vi "Display Right Click Menu.vi"(5 "Coords":T1, 7 "Tbl Refnum":refnum<vi>, 8 "error in (no error)":errorcluster, 9 "Menu Reference":refnum<k9>, 10 "Sync Notifier":refnum<notifier>, 11 "UserInterface in":refnum<class "UserInterface.lvclass">) -> (0 "error out":errorcluster)   [LabVIEW 2016, in "UserInterface.lvlib" / "UserInterface.lvclass"]
uses:
  UserInterface.lvclass
  <vilib>/Utility/miscctls.llb/LVPoint32TypeDef.ctl
  UserInterface.lvclass/UserInterface.ctl
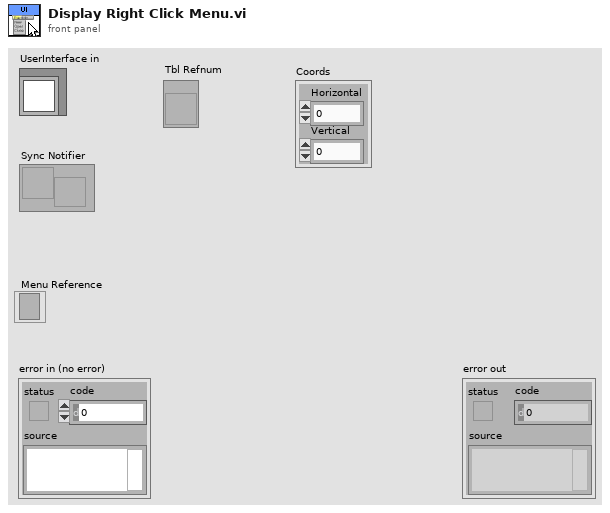
[diagram p1: front panel]
types:
  T1 = typedef "LVPoint32TypeDef.ctl" = cluster{"Horizontal":i32, "Vertical":i32}
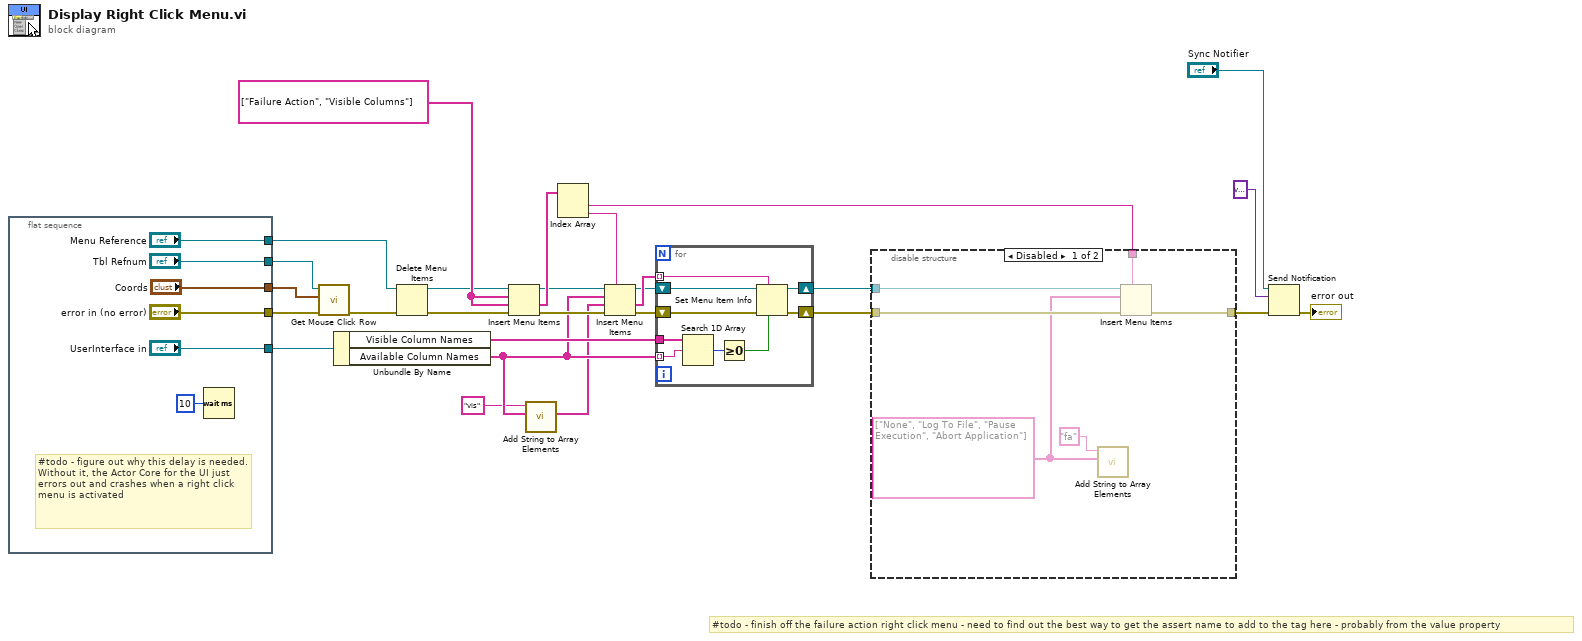
[diagram p0: block diagram]
diagram:
  w21 = string[] ["Failure Action", "Visible Columns"] ("item names")
  # "#todo - finish off the failure action right click menu - need to find out the best way to get the assert name to add to the tag here - probably from the value property"
  n1 = flat-sequence {
    tunnel: ["error in (no error)"] -> w27
    tunnel: ["UserInterface in"] -> w25
    tunnel: ["Menu Reference"] -> w8
    tunnel: ["Coords"] -> w5
    tunnel: ["Tbl Refnum"] -> w4
    frame #0 {
      # "#todo - figure out why this delay is needed. Without it, the Actor Core for the UI just errors out and crashes when a right click menu is activated"
      n2 = Wait (ms)(milliseconds to wait=u32 10) -> ()  [unwired: 1 out]
    }
  }
  n3 = call "Get Mouse Click Row.vi"("error in (no error)"=w27, "Coords"=w5, "Table in"=w4) -> ("error out"=w6:errorcluster)  [unwired: 5 in, 3 out]
  n4 = Unbundle By Name(w25) -> ("Visible Column Names"=w13:string[], "Available Column Names"=w12:string[])
  n5 = Delete Menu Items(6:w6, 9:w8) -> (0:w9:errorcluster, 3:w7:refnum<k9>)  [unwired: 2 in]
  n6 = Insert Menu Items(6:w9, 7:w21, 8:w21, 9:w7) -> (0:w26:errorcluster, 1:w19:string[], 3:w17:refnum<k9>)  [unwired: 2 in]
  n7 = call "Add String to Array Elements.vi"("String Array In"=w12, "Prepend String"="vis" ("string")) -> ("String Array Out"=w10:string[])  [unwired: 9 in]
  n8 = Index Array(array=w19) -> (element #1=w2:string, element #2=w18:string)  [unwired: 2 in]
  n9 = Insert Menu Items(5:w18, 6:w26, 7:w10, 8:w12, 9:w17) -> (0:w20:errorcluster, 1:w15:string[], 3:w14:refnum<k9>)  [unwired: 1 in]
  n10 = for {
    shift-right: [w41] -> w16
    shift-left: w20 -> [w42]
    tunnel: w15 -> [w40] mode=indexing
    tunnel: w13 -> [w38]
    tunnel: w12 -> [w37] mode=indexing
    shift-right: [w34] -> w1
    shift-left: w14 -> [w39]
    n11 = Search 1D Array(1D array=w38, element=w37) -> (index of element=w36:i32)  [unwired: 1 in]
    n12 = Greater Or Equal To 0?(x=w36) -> (x >= 0?=w35:bool)
    n13 = Set Menu Item Info(6:w35, 7:w40, 8:w42, 11:w39) -> (0:w41:errorcluster, 3:w34:refnum<k9>)  [unwired: 3 in]
  }
  n14 = disable-structure shown="Disabled" {
    disable-tunnel: w16 -> [w48 _]
    disable-tunnel: [w47 _] -> w3
    disable-tunnel: w2 -> [w46 _]
    disable-tunnel: w1 -> [w45 _]
    frame Disabled {
      w44 = string[] ["None", "Log To File", "Pause Execution", "Abort Application"]
      n15 = call "Add String to Array Elements.vi"("String Array In"=w44, "Prepend String"="fa") -> ()  [unwired: 9 in, 1 out]
      n16 = Insert Menu Items(5:w46, 6:w48, 8:w44, 9:w45) -> (0:w47:errorcluster)  [unwired: 2 in, 2 out]
    }
    frame Enabled {
    }
  }
  n17 = Send Notification(notification=variant, notifier="Sync Notifier", error in (no error)=w3) -> (error out=→"error out":errorcluster)  [unwired: 1 out]
